vi "Draw_Cage_Body.vi"(8 "error in (no error)":errorcluster, 9 "Cage type":T1 items=["Round", "Square", "Donut-maze", "T-maze", "Sociability maze", ""], 10 "Image Drawing Parameters":T2={"Draw Area Size"={"Width, pix"=480, "Height, pix"=480}, "Cage External Dims."={"Width, mm"=180.0, "Height, mm"=180.0}, "Background color"=13816530, "Image Scaling info"={"Fonts scale factor"=0.9603340292275574, "Pixels per mm"=2.5555555555555554}, "Segments Colors"={"Colors array for outer segments"=[14102567, 16625249, 14742520, 7646673, 16018755, 16703632, 11262441, 4552116, 6947347, 49913, 33129], "Colors array for midfield segments"=[8073876, 10935200, 34871, 12756431], "Color for central segment"=16777113, "Fill color for no segments image"=6316128}}, 11 "Refnum in":T7) -> (0 "error out":errorcluster, 3 "Refnum out":T7)   [LabVIEW 2018, in "Cage Diagram.lvlib"]
uses:
  Cage Diagram.lvlib
  <vilib>/vision/Image Controls.llb/IMAQ Image.ctl
  Typedefs/CTL_Cage_drawing_params.ctl
  SubVi's/Controls/CTL_Draw_Area_Size.ctl
  Typedefs/CTL_Cage_External_dimensions.ctl
  Typedefs/CTL_Image_Scaling_info.ctl
  SubVi's/Controls/CTL_Segments_Colors_(pie).ctl
  Typedefs/CTL_Cage_type.ctl
  Common_Resources.lvlib
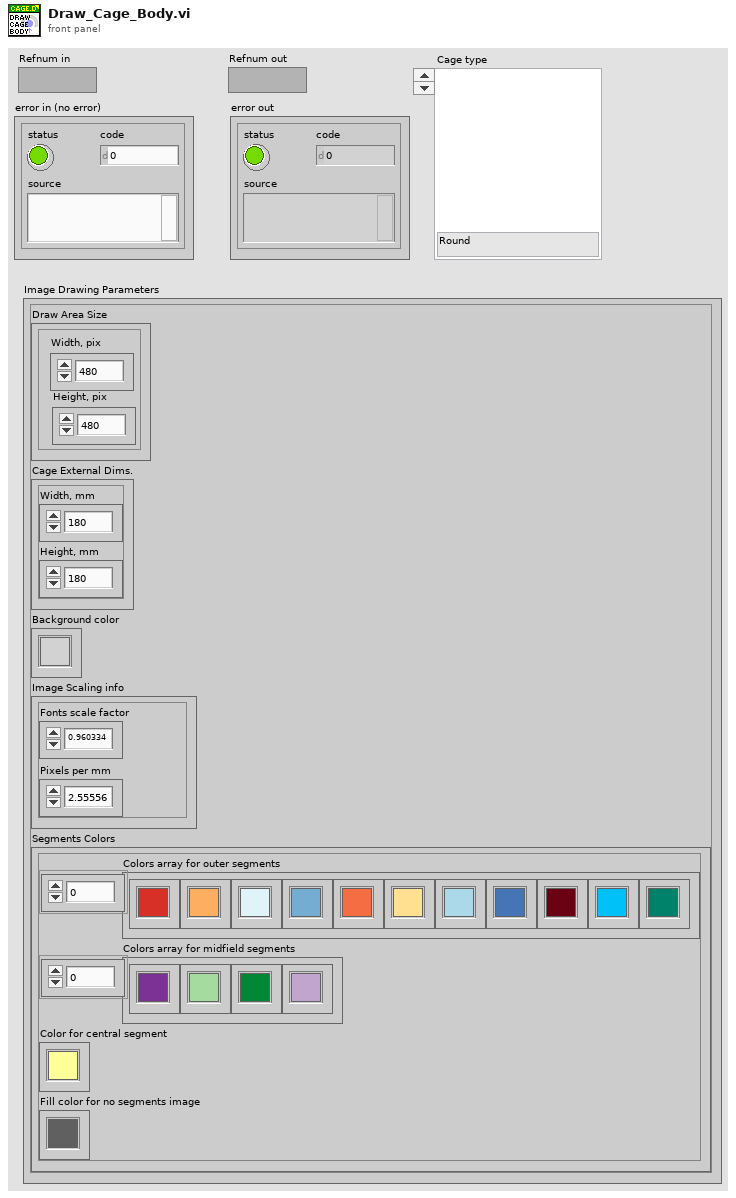
[diagram p1: front panel]
types:
  T1 = typedef "Cage Diagram.lvlib/CTL_Cage_type.ctl" = u16
  T2 = typedef "Cage Diagram.lvlib/CTL_Cage_drawing_params.ctl" = cluster{"Draw Area Size":T3, "Cage External Dims.":T4, "Background color":u32, "Image Scaling info":T5, "Segments Colors":T6}
  T3 = typedef "Common_Resources.lvlib/CTL_Draw_Area_Size.ctl" = cluster{"Width, pix":i32, "Height, pix":i32}
  T4 = typedef "Cage Diagram.lvlib/CTL_Cage_External_dimensions.ctl" = cluster{"Width, mm":dbl, "Height, mm":dbl}
  T5 = typedef "Cage Diagram.lvlib/CTL_Image_Scaling_info.ctl" = cluster{"Fonts scale factor":dbl, "Pixels per mm":dbl}
  T6 = typedef "Common_Resources.lvlib/CTL_Segments_Colors_(pie).ctl" = cluster{"Colors array for outer segments":u32[], "Colors array for midfield segments":u32[], "Color for central segment":u32, "Fill color for no segments image":u32}
  T7 = typedef "IMAQ Image.ctl" = refnum<image>
  T8 = cluster{"X Left":dbl, "Y Top":dbl, "X Right":dbl, "Y Bottom":dbl}
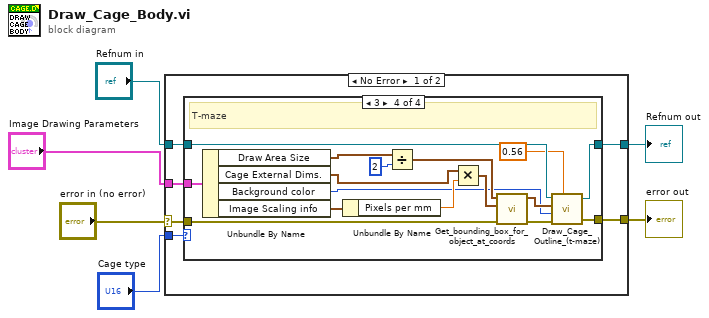
[diagram p0: block diagram]
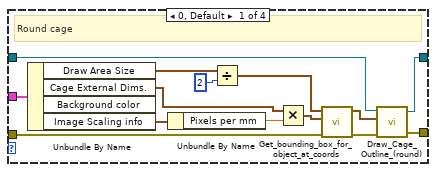
[diagram p2: hidden frame]
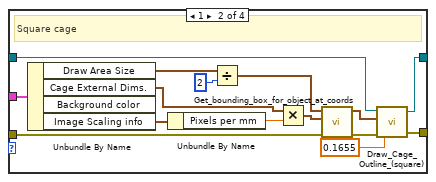
[diagram p3: hidden frame]
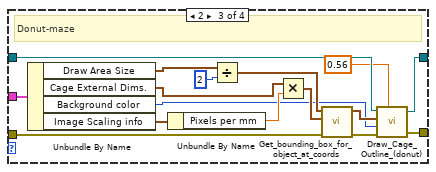
[diagram p4: hidden frame]
diagram:
  n1 = case shown="No Error" "error in (no error)" {
    selector: "error in (no error)" -> [w8 w75]
    tunnel: [w9 w75] -> w5
    tunnel: "Refnum in" -> [w10 w74]
    tunnel: "Image Drawing Parameters" -> [w7 _]
    tunnel: [w11 w74] -> w2
    tunnel: "Cage type" -> [w12 _]
    frame No Error {
      n2 = case shown="3" w12 {
        tunnel: [w13 w28 w44 w60] -> w11
        tunnel: w10 -> [w14 w29 w45 w61]
        tunnel: [w16 w31 w47 w63] -> w9
        tunnel: w8 -> [w18 w33 w49 w65]
        tunnel: w7 -> [w26 w41 w57 w73]
        frame 0, Default {
          # "Round cage"
          n3 = Unbundle By Name(w26) -> ("Draw Area Size"=w25:T3, "Cage External Dims."=w22:T4, "Image Scaling info"=w20:T5)  [unwired: 1 out]
          n4 = Unbundle By Name(w20) -> ("Pixels per mm"=w19:dbl)
          n5 = Divide(x=w25, y=2) -> (x/y=w23:cluster{"Width, pix":dbl, "Height, pix":dbl})
          n6 = Multiply(x=w22, y=w19) -> (x*y=w21:T4)
          n7 = call "Get_bounding_box_for_object_at_coords.vi"("Error In"=w18, "Object Size, pix"=w21, "Object Coords, pix"=w23) -> ("Error Out"=w17:errorcluster, "Object Bounding Box"=w15:T8)  [unwired: 7 in]
          n8 = call "Draw_Cage_Outline_(round).vi"("Error In"=w17, "Bounding rectangle for cage outline, pix"=w15, "Picture refnum in"=w14) -> ("Error Out"=w16:errorcluster, "Picture refnum out"=w13:T7)  [unwired: 2 in]
        }
        frame 1 {
          # "Square cage"
          n9 = Unbundle By Name(w41) -> ("Draw Area Size"=w40:T3, "Cage External Dims."=w37:T4, "Image Scaling info"=w35:T5)  [unwired: 1 out]
          n10 = Unbundle By Name(w35) -> ("Pixels per mm"=w34:dbl)
          n11 = Divide(x=w40, y=2) -> (x/y=w38:cluster{"Width, pix":dbl, "Height, pix":dbl})
          n12 = Multiply(x=w37, y=w34) -> (x*y=w36:T4)
          n13 = call "Get_bounding_box_for_object_at_coords.vi"("Error In"=w33, "Object Size, pix"=w36, "Object Coords, pix"=w38) -> ("Error Out"=w32:errorcluster, "Object Bounding Box"=w30:T8)  [unwired: 7 in]
          n14 = call "Draw_Cage_Outline_(square).vi"("Error In"=w32, "Corner scale  factor"=0.1655, "Bounding rectangle for cage outline, pix"=w30, "Picture refnum in"=w29) -> ("Error Out"=w31:errorcluster, "Picture refnum out"=w28:T7)  [unwired: 1 in]
        }
        frame 2 {
          # "Donut-maze"
          n15 = Unbundle By Name(w57) -> ("Draw Area Size"=w56:T3, "Cage External Dims."=w53:T4, "Background color"=w43:u32, "Image Scaling info"=w51:T5)
          n16 = Unbundle By Name(w51) -> ("Pixels per mm"=w50:dbl)
          n17 = Divide(x=w56, y=2) -> (x/y=w54:cluster{"Width, pix":dbl, "Height, pix":dbl})
          n18 = Multiply(x=w53, y=w50) -> (x*y=w52:T4)
          n19 = call "Get_bounding_box_for_object_at_coords.vi"("Error In"=w49, "Object Size, pix"=w52, "Object Coords, pix"=w54) -> ("Error Out"=w48:errorcluster, "Object Bounding Box"=w46:T8)  [unwired: 7 in]
          n20 = call "Draw_Cage_Outline_(donut).vi"("Picture refnum in"=w45, "Bounding rectangle for cage outline, pix"=w46, "Background color"=w43, "Error In"=w48, "Inner donut scale factor"=0.56) -> ("Picture refnum out"=w44:T7, "Error Out"=w47:errorcluster)  [unwired: 1 in]
        }
        frame 3 {
          # "T-maze"
          n21 = Unbundle By Name(w73) -> ("Draw Area Size"=w72:T3, "Cage External Dims."=w69:T4, "Background color"=w59:u32, "Image Scaling info"=w67:T5)
          n22 = Unbundle By Name(w67) -> ("Pixels per mm"=w66:dbl)
          n23 = Divide(x=w72, y=2) -> (x/y=w70:cluster{"Width, pix":dbl, "Height, pix":dbl})
          n24 = Multiply(x=w69, y=w66) -> (x*y=w68:T4)
          n25 = call "Get_bounding_box_for_object_at_coords.vi"("Error In"=w65, "Object Size, pix"=w68, "Object Coords, pix"=w70) -> ("Error Out"=w64:errorcluster, "Object Bounding Box"=w62:T8)  [unwired: 7 in]
          n26 = call "Draw_Cage_Outline_(t-maze).vi"("Picture refnum in"=w61, "Bounding rectangle for cage outline, pix"=w62, "Background color"=w59, "Error In"=w64, "Inner donut scale factor"=0.56) -> ("Picture refnum out"=w60:T7, "Error Out"=w63:errorcluster)  [unwired: 1 in]
        }
      }
    }
    frame Error {
    }
  }
  "Refnum out" <- w2
  "error out" <- w5
